vi "updateDeviceStatus.vi"(8 "error in (no error)":errorcluster, 10 "isNewData":bool, 11 "Orion_BMS in":refnum<class "Orion_BMS.lvclass">) -> (0 "error out":errorcluster, 3 "Orion_BMS out":refnum<class "Orion_BMS.lvclass">)   [LabVIEW 2017, in "Orion_BMS.lvclass"]
doc: "Used whether there is recent reads in the TPDO data to determine whether the device is responsive or not"
uses:
  Orion_BMS.lvclass
  Orion_BMS.lvclass/Orion_BMS.ctl
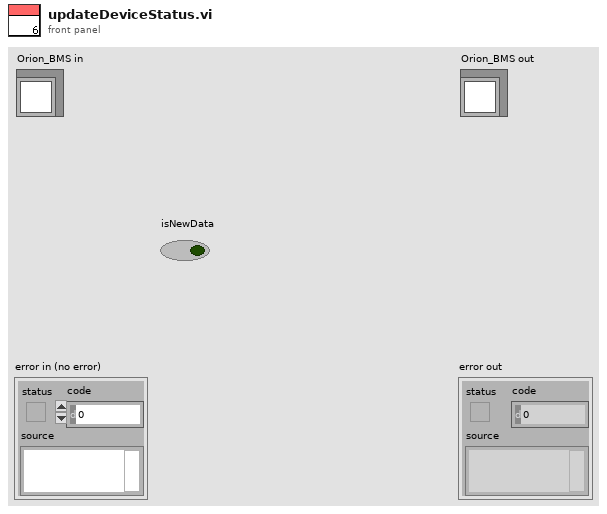
[diagram p1: front panel]
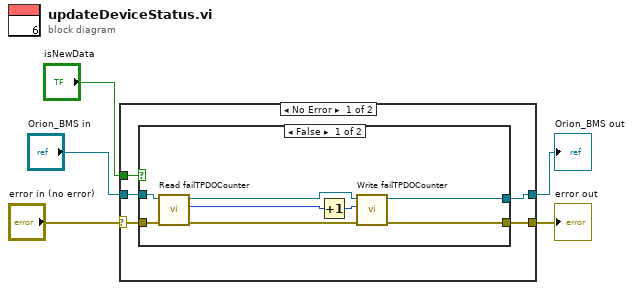
[diagram p0: block diagram]
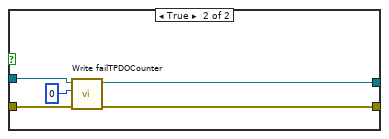
[diagram p2: hidden frame]
diagram:
  n1 = case shown="No Error" "error in (no error)" {
    selector: "error in (no error)" -> [w8 w25]
    tunnel: [w6 w25] -> w4
    tunnel: [w7 w24] -> w2
    tunnel: "Orion_BMS in" -> [w9 w24]
    tunnel: "isNewData" -> [w10 _]
    frame No Error {
      n2 = case shown="False" w10 {
        tunnel: w9 -> [w18 w23]
        tunnel: w8 -> [w17 w21]
        tunnel: [w12 w20] -> w7
        tunnel: [w11 w19] -> w6
        frame False {
          n3 = call "Read failTPDOCounter.vi"("error in (no error)"=w17, "Orion_BMS in"=w18) -> ("error out"=w14:errorcluster, "failTPDOCounter"=w16:u32, "Orion_BMS out"=w13:refnum<class "Orion_BMS.lvclass">)  [unwired: 7 in]
          n4 = Increment(x=w16) -> (x+1=w15:u32)
          n5 = call "Write failTPDOCounter.vi"("error in (no error)"=w14, "failTPDOCounter"=w15, "Orion_BMS in"=w13) -> ("error out"=w11:errorcluster, "Orion_BMS out"=w12:refnum<class "Orion_BMS.lvclass">)  [unwired: 7 in]
        }
        frame True {
          n6 = call "Write failTPDOCounter.vi"("error in (no error)"=w21, "failTPDOCounter"=u32 0, "Orion_BMS in"=w23) -> ("error out"=w19:errorcluster, "Orion_BMS out"=w20:refnum<class "Orion_BMS.lvclass">)  [unwired: 7 in]
        }
      }
    }
    frame Error {
    }
  }
  "error out" <- w4
  "Orion_BMS out" <- w2
